vi "Get Routing Channel Configuration.vi"(8 "error in":errorcluster, 11 "routing channel in":T1 format="%.0x") -> (0 "error out":errorcluster, 1 "state configurations":T2, 2 "routing channel name":string, 3 "routing channel out":T1 format="%.0x", 4 "initial state":string, 6 "description":string)   [LabVIEW 2020, in "Routing and Faulting Scripting.lvlib"]
doc: "Returns the name, description, and state configuration of a specified routing channel."
uses:
  Routing and Faulting Scripting.lvlib
  <vilib>/NI VeriStand/Custom Device API/Custom Device Item Ref.ctl
  Shared/Channel States.ctl
  Shared/Routing State.ctl
  Shared/Connection.ctl
  <vilib>/NI VeriStand/Custom Device API/Custom Device API.lvlib
  Shared/Routing and Faulting Shared.lvlib
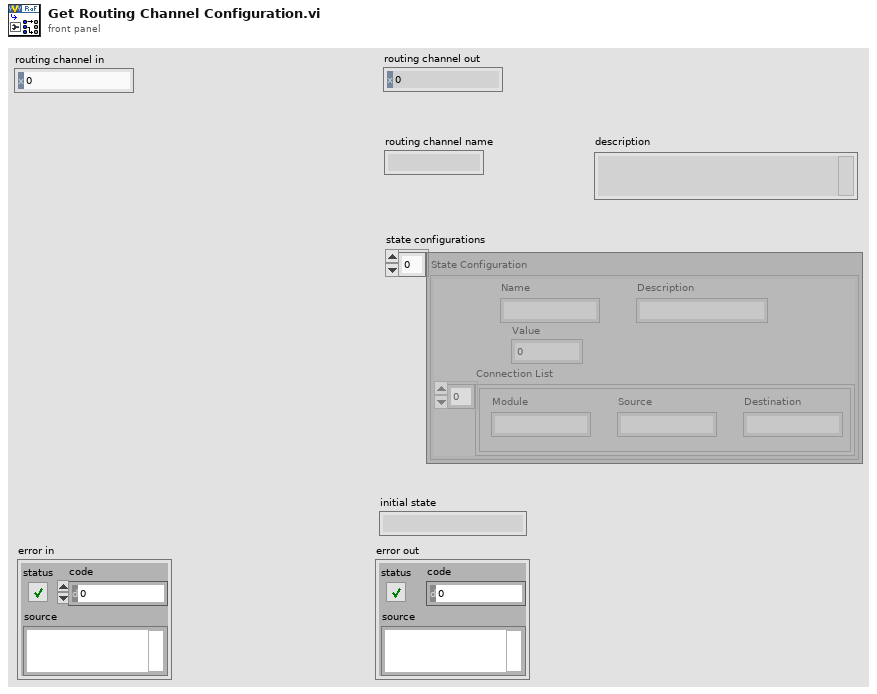
[diagram p1: front panel]
types:
  T1 = typedef "Custom Device API.lvlib/Custom Device Item Ref.ctl" = u64
  T2 = typedef "Routing and Faulting Shared.lvlib/Channel States.ctl" = T3[]
  T3 = typedef "Routing and Faulting Shared.lvlib/Routing State.ctl" = cluster{"Name":string, "Description":string, "Value":i32, "Connection List":T4[]}
  T4 = typedef "Routing and Faulting Shared.lvlib/Connection.ctl" = cluster{"Module":string, "Source":string, "Destination":string}
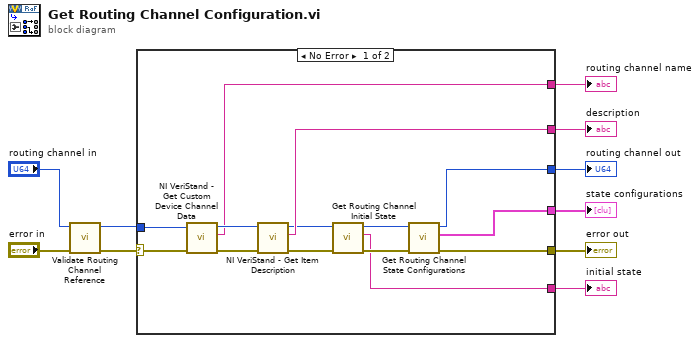
[diagram p0: block diagram]
diagram:
  n1 = call "Validate Routing Channel Reference.vi"("error in"="error in", "routing channel in"="routing channel in") -> ("error out"=w3:errorcluster, "routing channel out"=w1:T1)  [unwired: 8 in]
  n2 = case shown="No Error" w3 {
    selector: w3 -> [w24 w25]
    tunnel: [w22 w25] -> w10
    tunnel: w1 -> [w21 _]
    tunnel: [w17 _] -> w7
    tunnel: [w23 _] -> w8
    tunnel: [w20 _] -> w6
    tunnel: [w16 _] -> w5
    tunnel: [w11 _] -> w4
    frame No Error {
      n3 = call <vilib>:"NI VeriStand - Get Custom Device Channel Data.vi"("error in (no error)"=w24, "Channel Ref in"=w21) -> ("error out"=w18:errorcluster, "Channel Name"=w17:string, "Channel Ref out"=w19:T1)  [unwired: 4 in, 3 out]
      n4 = call <vilib>:"NI VeriStand - Get Item Description.vi"("error in (no error)"=w18, "Item Ref in"=w19) -> ("error out"=w13:errorcluster, "Description"=w16:string, "Item Ref out"=w15:T1)  [unwired: 6 in, 1 out]
      n5 = call "Get Routing Channel Initial State.vi"("error in"=w13, "routing channel in"=w15) -> ("error out"=w12:errorcluster, "initial state"=w11:string, "routing channel out"=w14:T1)  [unwired: 7 in]
      n6 = call "Get Routing Channel State Configurations.vi"("error in"=w12, "routing channel in"=w14) -> ("error out"=w22:errorcluster, "state configurations"=w23:T2, "routing channel out"=w20:T1)  [unwired: 7 in]
    }
    frame Error {
    }
  }
  "error out" <- w10
  "routing channel name" <- w7
  "state configurations" <- w8
  "routing channel out" <- w6
  "description" <- w5
  "initial state" <- w4
